vi "Sequence.BuildMain.vi"(6 "Iterations":u32, 8 "error in (no error)":errorcluster, 9 "Sequence Channels":T1, 10 "Steps":T3[](array[typedef]), 11 "Sequence":refnum<k24>) -> (0 "error out":errorcluster, 3 "Sequence out":refnum<k24>)   [LabVIEW 2015, in "Single Station Execution.lvlib"]
uses:
  Single Station Execution.lvlib
  NationalInstruments.VeriStand.RealTimeSequenceDefinitionApi
  Types/Compiled.StepProperties.ctl
  Types/Compiled.IOStateProperties.ctl
  Types/Compiled.StepElementProperties.ctl
  Types/Channel.Properties.ctl
  Types/Step.Types.ctl
  Types/Compiled.StepCondition.ctl
  Types/Conditions.OperationTypes.ctl
  Types/Compiled.SequenceChannels.ctl
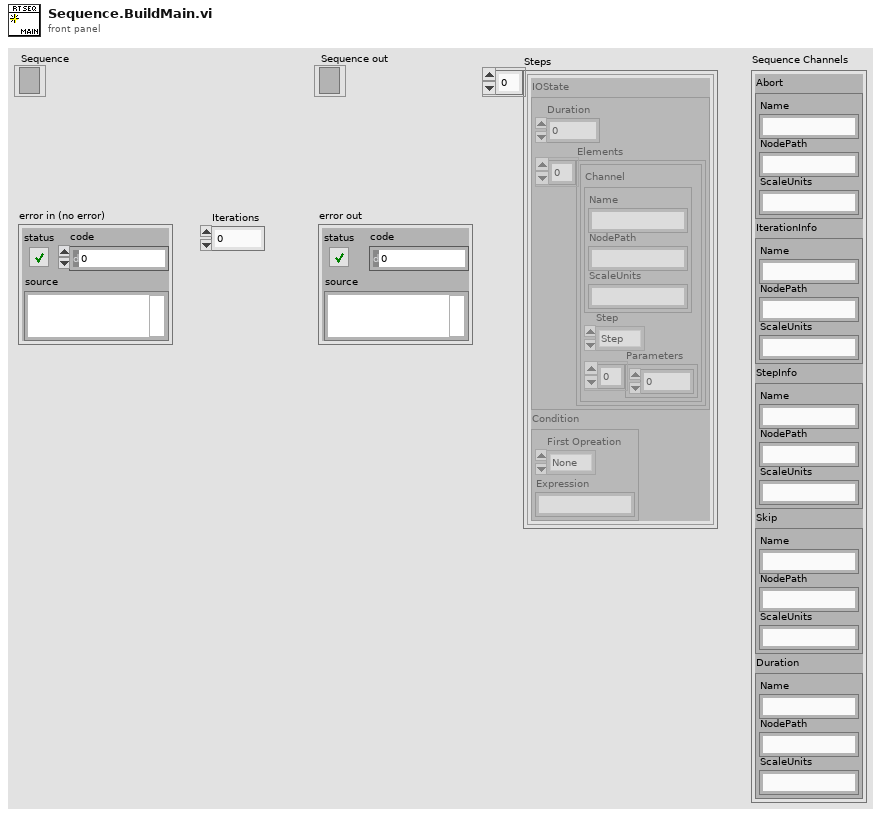
[diagram p1: front panel]
types:
  T1 = typedef "Single Station Execution.lvlib/Compiled.SequenceChannels.ctl" = cluster{"Abort":T2, "IterationInfo":T2, "StepInfo":T2, "Skip":T2, "Duration":T2}
  T2 = typedef "Single Station Execution.lvlib/Channel.Properties.ctl" = cluster{"Name":string, "NodePath":string, "ScaleUnits":string}
  T3 = typedef "Single Station Execution.lvlib/Compiled.StepProperties.ctl" = cluster{"IOState":T4, "Condition":T7}
  T4 = typedef "Single Station Execution.lvlib/Compiled.IOStateProperties.ctl" = cluster{"Duration":dbl, "Elements":T5[]}
  T5 = typedef "Single Station Execution.lvlib/Compiled.StepElementProperties.ctl" = cluster{"Channel":T2, "Step":T6, "Parameters":dbl[]}
  T6 = typedef "Single Station Execution.lvlib/Step.Types.ctl" = enum8{"Step", "iStep", "Ramp", "Unchanged", "Unknown", "Sine", "LogSine", "LinearSine", "ForcedRamp", "Waveform"}
  T7 = typedef "Single Station Execution.lvlib/Compiled.StepCondition.ctl" = cluster{"First Opreation":T8, "Expression":string}
  T8 = typedef "Single Station Execution.lvlib/Conditions.OperationTypes.ctl" = enum8{"None", "&&", "||"}
  T9 = typedef "Single Station Execution.lvlib/Sequence.MainSeqRefs.ctl" = cluster{"Task.Main":refnum<k24>, "For.Main":refnum<k24>, "While.Main":refnum<k24>, "SelectCases.Main":refnum<k24>, "Switch.Main":refnum<k24>}
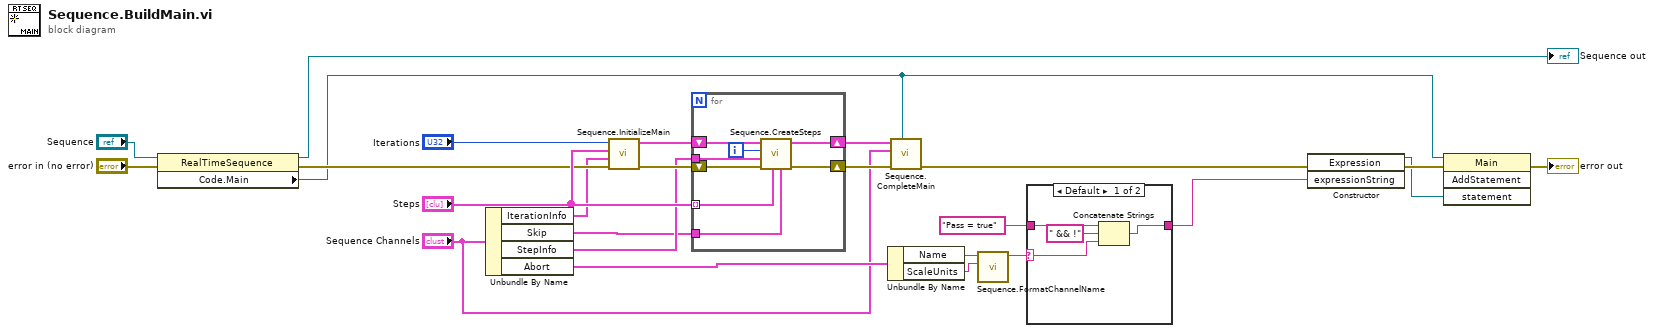
[diagram p0: block diagram]
diagram:
  n1 = property class="RealTimeSequence"(reference="Sequence", error in="error in (no error)") -> (reference out=→"Sequence out":refnum<k24>, error out=w19:errorcluster, "Code.Main"=w8:refnum<k24>)
  n2 = Unbundle By Name("Sequence Channels") -> ("IterationInfo"=w17:T2, "Skip"=w13:T2, "StepInfo"=w15:T2, "Abort"=w6:T2)
  n3 = call "Sequence.InitializeMain.vi"("error in (no error)"=w19, "IterationInfo"=w17, "Steps"="Steps", "Iterations"="Iterations") -> ("error out"=w22:errorcluster, "Refs"=w16:T9)  [unwired: 6 in]
  n4 = for {
    tunnel: "Steps" -> [w27] mode=indexing
    shift-right: [w33] -> w23
    shift-left: w22 -> [w30]
    tunnel: w15 -> [w31]
    shift-right: [w28] -> w14
    shift-left: w16 -> [w29]
    tunnel: w13 -> [w26]
    i -> [w32]
    n5 = call "Sequence.CreateSteps.vi"("Skip"=w26, "Step"=w27, "error in (no error)"=w30, "StepInfo"=w31, "Iteration"=w32, "Refs"=w29) -> ("error out"=w33:errorcluster, "Refs out"=w28:T9)  [unwired: 4 in]
  }
  n6 = Unbundle By Name(w6) -> ("Name"=w5:string, "ScaleUnits"=w4:string)
  n7 = call "Sequence.CompleteMain.vi"("Code.Main"=w8, "error in (no error)"=w23, "Sequence Channels"="Sequence Channels", "Refs"=w14) -> ("error out"=w11:errorcluster)  [unwired: 7 in]
  n8 = call "Sequence.FormatChannelName.vi"("ScaleUnits"=w4, "Name"=w5) -> ("ChannelName"=w3:string)  [unwired: 9 in]
  n9 = case shown="Default" w3 {
    selector: w3 -> [w35 _]
    tunnel: [w34 w38] -> w7
    tunnel: "Pass = true" ("expressionString") -> [w37 w38]
    frame Default {
      n10 = Concatenate Strings(w37, " && !" ("string"), w35) -> (w34:string)
    }
    frame "" {
    }
  }
  n11 = constructor class="Expression"(error in=w11, "expressionString"=w7) -> (reference out=w9:refnum<k24>, error out=w10:errorcluster)  [unwired: 2 in, 2 out]
  n12 = invoke class="Main" method="AddStatement"(reference=w8, error in=w10, "statement"=w9) -> (error out=→"error out":errorcluster)  [unwired: 1 in, 3 out]
